vi "SendMultiPacketRetry.vi"(7 "Num Retries":i32=3, 8 "error in (no error)":errorcluster, 9 "PIDIn":u8, 10 "Packets In":T1[](array[typedef]), 11 "VISA resource name":refnum<visa-resource-name>) -> (0 "error out":errorcluster, 1 "PIDOut":u8, 2 "Packets Out":T1[](array[typedef]), 3 "VISA resource name 2":refnum<visa-resource-name>)   [LabVIEW 2009]
uses:
  Packet.ctl
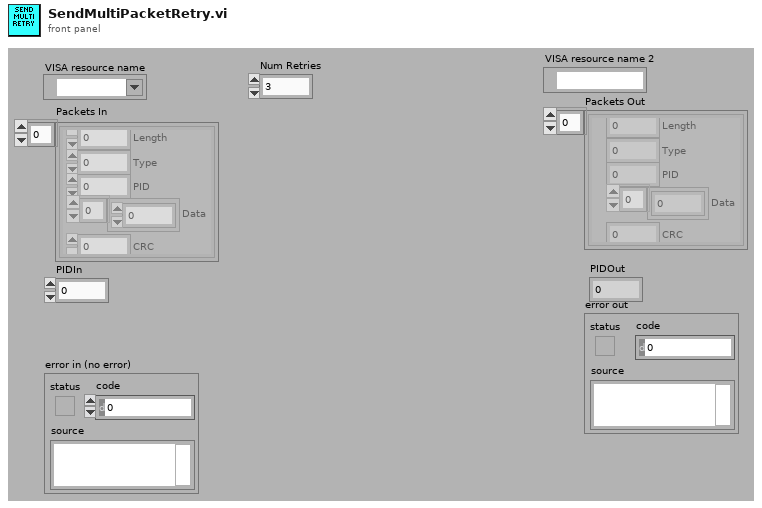
[diagram p1: front panel]
types:
  T1 = typedef "Packet.ctl" = cluster{"Length":u8, "Type":u8, "PID":u8, "Data":u8[], "CRC":u8}
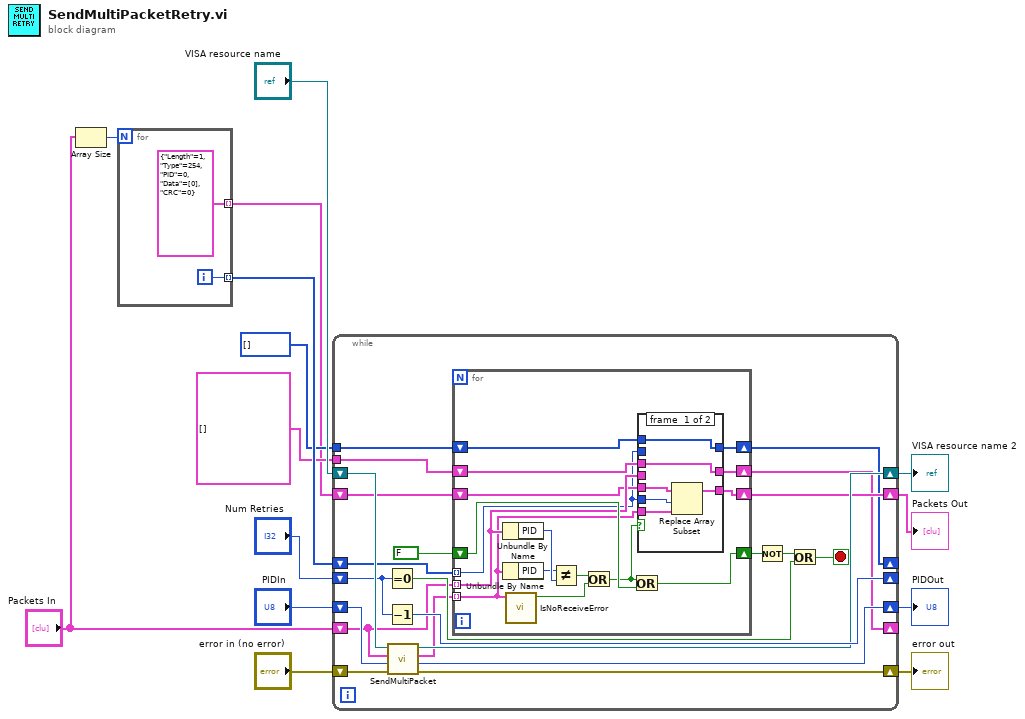
[diagram p0: block diagram]
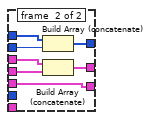
[diagram p2: hidden frame]
diagram:
  n1 = Array Size(array="Packets In") -> (size(s)=w2:i32)
  n2 = for {
    N: w2 -> [_]
    tunnel: [w16] -> w6 mode=indexing
    tunnel: [T1 {"Length"=1, "Type"=254, "PID"=0, "Data"=[0], "CRC"=0} ("Transmit")] -> w1 mode=indexing
    i -> [w16]
  }
  n3 = while {
    shift-right: [w31] -> w10
    shift-left: "error in (no error)" -> [w37]
    shift-right: [w32] -> w11
    shift-left: "VISA resource name" -> [w38]
    shift-right: [w35] -> _
    shift-left: "Num Retries" -> [w34]
    shift-right: [w21] -> _
    shift-left: "Packets In" -> [w24]
    shift-right: [w25] -> w8
    shift-left: w1 -> [w26]
    shift-right: [w30] -> w3
    shift-left: "PIDIn" -> [w29]
    shift-right: [w20] -> _
    shift-left: w6 -> [w27]
    tunnel: i32[] [] ("Data") -> [w23]
    tunnel: T1[] [] -> [w22]
    stop <- w33 stop-if-true
    n4 = Equal To 0?(x=w34) -> (x = 0?=w36:bool)
    n5 = Decrement(x=w34) -> (x-1=w35:i32)
    n6 = call "SendMultiPacket.vi"("error in (no error)"=w37, "PIDIn"=w29, "Packets In"=w24, "VISA resource name"=w38) -> ("error out"=w31:errorcluster, "PIDOut"=w30:u8, "ReceivedBytes"=w28:T1[], "VISA resource name out"=w32:refnum<visa-resource-name>)  [unwired: 4 in]
    n7 = for {
      tunnel: w28 -> [w40] mode=indexing
      tunnel: w27 -> [w41] mode=indexing
      shift-right: [w39] -> w25
      shift-left: w26 -> [w42]
      tunnel: w24 -> [w48] mode=indexing
      shift-right: [w52] -> w21
      shift-left: w22 -> [w53]
      shift-right: [w51] -> w20
      shift-left: w23 -> [w54]
      shift-right: [w49] -> w17
      shift-left: FALSE ("IsNotReceived?") -> [w50]
      n8 = Unbundle By Name(w48) -> ("PID"=w47:u8)
      n9 = Unbundle By Name(w40) -> ("PID"=w46:u8)
      n10 = call "IsNoReceiveError.vi"("Packet"=w40) -> ("IsNotReceived?"=w44:bool)  [unwired: 10 in]
      n11 = Not Equal?(x=w46, y=w47) -> (x != y?=w43:bool)
      n12 = Or(x=w43, y=w44) -> (x .or. y?=w45:bool)
      n13 = Or(x=w45, y=w50) -> (x .or. y?=w49:bool)
      n14 = case shown="True" w45 {
        tunnel: w48 -> [_ w66]
        tunnel: w41 -> [_ w64]
        tunnel: w54 -> [w60 w65]
        tunnel: w53 -> [w59 w67]
        tunnel: [w59 w63] -> w52
        tunnel: [w60 w62] -> w51
        tunnel: w42 -> [w58 w61]
        tunnel: w41 -> [w57 _]
        tunnel: w40 -> [w56 _]
        tunnel: [w55 w61] -> w39
        frame #0 {
          n15 = Replace Array Subset(array=w58, new element=w56, index=w57) -> (w55:T1[])
        }
        frame #1 {
          n16 = Build Array (concatenate)(w65, w64) -> (w62:i32[])
          n17 = Build Array (concatenate)(w67, w66) -> (w63:T1[])
        }
      }
    }
    n18 = Not(x=w17) -> (.not. x?=w18:bool)
    n19 = Or(x=w18, y=w36) -> (x .or. y?=w33:bool)
  }
  "VISA resource name 2" <- w11
  "Packets Out" <- w8
  "error out" <- w10
  "PIDOut" <- w3
